vi "ReadBytesAtPort.vi"(8 "Error In":errorcluster, 11 "Sierra M100 In":refnum<visa-resource-name>) -> (0 "Error Out":errorcluster, 2 "Read Buffer":string, 3 "Sierra M100 Out":refnum<visa-resource-name>)   [LabVIEW 2012, in "Sierra-M100.lvlib"]
doc: "This VI reads the bytes at the serial port and flushes the receive buffer after reading. There is 100 msec wait before reading all of the bytes."
uses:
  Sierra-M100.lvlib
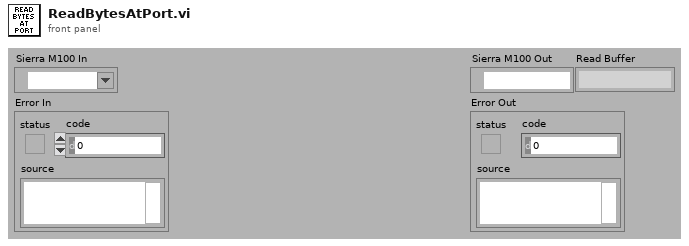
[diagram p1: front panel]
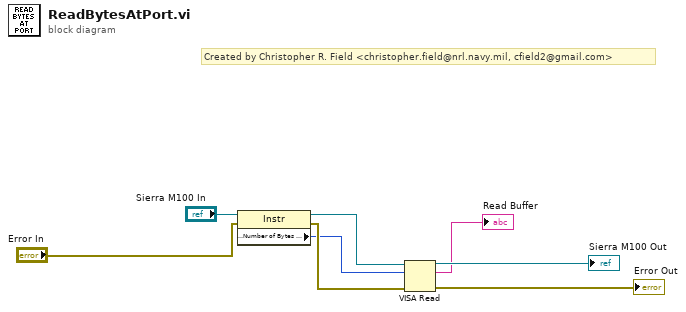
[diagram p0: block diagram]
diagram:
  # "Created by Christopher R. Field <christopher.field@nrl.navy.mil, cfield2@gmail.com>"
  n1 = property class="Instr"(reference="Sierra M100 In", error in="Error In") -> (reference out=w8:refnum<visa-resource-name>, error out=w7:errorcluster, "Serial Settings:Number of Bytes at Serial Port"=w6:u32)
  n2 = VISA Read(VISA resource name=w8, byte count=w6, error in (no error)=w7) -> (VISA resource name out=→"Sierra M100 Out":refnum<visa-resource-name>, read buffer=→"Read Buffer":string, error out=→"Error Out":errorcluster)  [unwired: 1 out]
